vi "GPIO Number.vi"(4 "PWM in":refnum<class "PWM.lvclass">) -> (7 "GPIO #":T1=-1)   [LabVIEW 2024, in "CTI.lvlib" / "PWM.lvclass"]
uses:
  PWM.lvclass
  GPIO Number.ctl
  PWM.lvclass/PWM.ctl
  CTI.lvlib
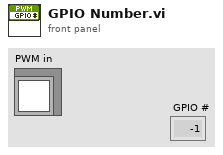
[diagram p1: front panel]
types:
  T1 = typedef "CTI.lvlib/GPIO Number.ctl" = i8
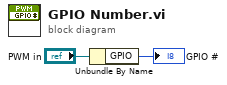
[diagram p0: block diagram]
diagram:
  n1 = Unbundle By Name("PWM in") -> ("GPIO"=→"GPIO #":T1)
